vi "Init Events.vi"(8 "error in (no error)":errorcluster, 11 "LV Chat Server in":refnum<class "LV Chat Server.lvclass">) -> (0 "error out":errorcluster, 3 "LV Chat Server out":refnum<class "LV Chat Server.lvclass">)   [LabVIEW 2020, in "LV Chat Server.lvclass"]
uses:
  LV Chat Server.lvclass
  Stream-Simple-Msg/Endpoint/Endpoint.lvclass
  Log Event Data.ctl
  Data Types/Message.ctl
  LV Chat Server.lvclass/LV Chat Server.ctl
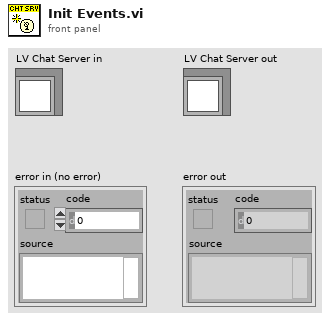
[diagram p1: front panel]
types:
  T1 = typedef "LV Chat Server.lvclass/Log Event Data.ctl" = cluster{"Item":T2}
  T2 = typedef "Message.ctl" = cluster{"From":string, "Time":dbl, "Message":string}
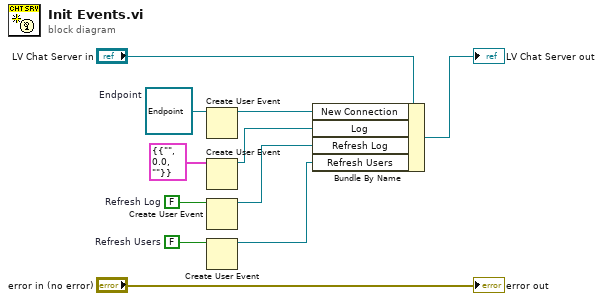
[diagram p0: block diagram]
diagram:
  w2 = FALSE  # Refresh Users
  w4 = FALSE  # Refresh Log
  w8 = refnum<class "Endpoint.lvclass"> refnum  # Endpoint
  n1 = Create User Event(user event datatype=w8) -> (user event=w7:refnum<user-event>)  [unwired: 1 in, 1 out]
  n2 = Create User Event(user event datatype=T1 {"Item"={"From"="", "Time"=0.0, "Message"=""}} ("Log Event Data")) -> (user event=w5:refnum<user-event>)  [unwired: 1 in, 1 out]
  n3 = Create User Event(user event datatype=w4) -> (user event=w3:refnum<user-event>)  [unwired: 1 in, 1 out]
  n4 = Create User Event(user event datatype=w2) -> (user event=w1:refnum<user-event>)  [unwired: 1 in, 1 out]
  n5 = Bundle By Name(cluster="LV Chat Server in", "New Connection"=w7, "Log"=w5, "Refresh Log"=w3, "Refresh Users"=w1) -> (→"LV Chat Server out":refnum<class "LV Chat Server.lvclass">)
  "error out" <- "error in (no error)"
